vi "testBasic Root Folder Example.vi"(8 "error in (no error)":errorcluster, 11 "TestCase in":refnum<class "Calculate Output Directory Tests.lvclass">) -> (0 "error out":errorcluster, 3 "TestCase out":refnum<class "Calculate Output Directory Tests.lvclass">)   [LabVIEW 2014, in "Calculate Output Directory Tests.lvclass"]
uses:
  Calculate Output Directory Tests.lvclass
  <vilib>/addons/_JKI Toolkits/VI Tester/TestCase.llb/TestCase.lvclass
  G CLI LvBuild.lvlib
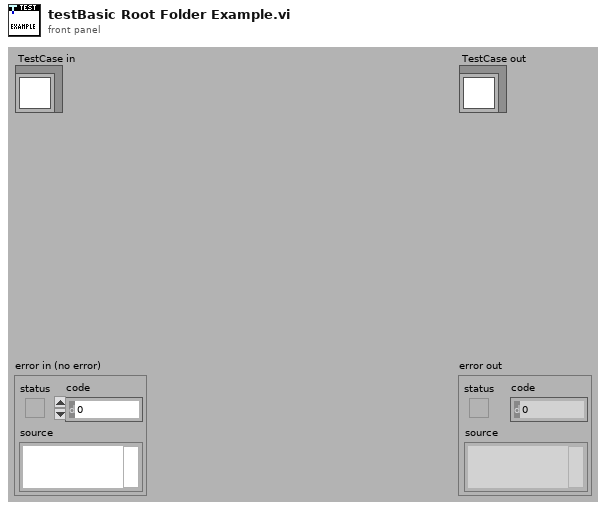
[diagram p1: front panel]
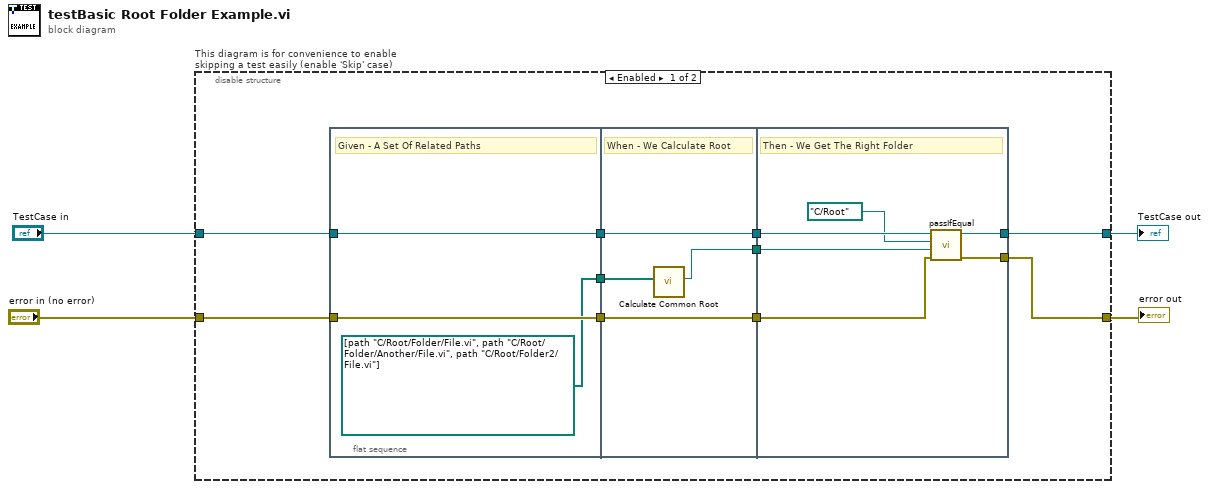
[diagram p0: block diagram]
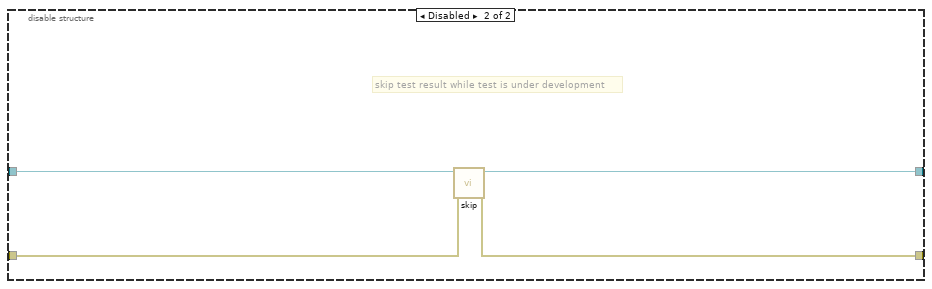
[diagram p2: hidden frame]
diagram:
  n1 = disable-structure "This diagram is for convenience to enable skipping a test easily (enable 'Skip' case)" shown="Enabled" {
    disable-tunnel: "TestCase in" -> [w11 w31]
    disable-tunnel: [w14 w29] -> w1
    disable-tunnel: [w10 w30] -> w3
    disable-tunnel: "error in (no error)" -> [w7 w28]
    frame Enabled {
      n2 = flat-sequence {
        tunnel: [w17] -> w12
        tunnel: w11 -> [w17]
        tunnel: [w16] -> w8
        tunnel: w7 -> [w16]
        tunnel: [path[] [path "C:/Root/Folder/File.vi", path "C:/Root/Folder/Another/File.vi", path "C:/Root/Folder2/File.vi"] ("Generated Files")] -> w5
        tunnel: [w21] -> w13
        tunnel: w12 -> [w21]
        tunnel: [w20] -> w9
        tunnel: w8 -> [w20]
        tunnel: [w19] -> w6
        tunnel: w5 -> [w18]
        tunnel: [w27] -> w14
        tunnel: w13 -> [w26]
        tunnel: [w25] -> w10
        tunnel: w9 -> [w24]
        tunnel: w6 -> [w23]
        frame #0 {
          # "Given - A Set Of Related Paths"
        }
        frame #1 {
          # "When - We Calculate Root"
          n3 = call "Calculate Common Root.vi"("Generated Files"=w18) -> ("Root Path"=w19:path)  [unwired: 9 in, 1 out]
        }
        frame #2 {
          # "Then - We Get The Right Folder"
          n4 = call-dynamic "passIfEqual.vi"("error in (no error)"=w24, "y"=w23, "x"=path "C:/Root" ("Root Path"), "TestCase in"=w26) -> ("error out"=w25:errorcluster, "TestCase out"=w27:refnum<class "Calculate Output Directory Tests.lvclass">)  [unwired: 6 in]
        }
      }
    }
    frame Disabled {
      # "skip test result while test is under development"
      n5 = call <vilib>:"skip.vi"("error in (no error)"=w28, "TestCase in"=w31) -> ("error out"=w30:errorcluster, "TestCase out"=w29:refnum<class "Calculate Output Directory Tests.lvclass">)  [unwired: 8 in]
    }
  }
  "error out" <- w3
  "TestCase out" <- w1
